vi "Main_Taper.vi"() -> ()   [LabVIEW 2016]
uses:
  <vilib>/Instr/_visa.llb/VISA Configure Serial Port (Instr).vi
panel:
  in  "Tab Control":T1(tab)=enum."Taper Time"
  in  "Stop Taper":bool
  out "COM_OK":bool
  in  "Send":bool
  in  "Start":bool
  in  "COM Write":string="AA;\nVL10.0000;\nAX;\nLS20;\nMR4.0000;\nGO;\nMR-4.0000;\nGO;\nLE;\nAA;\nVL1.0000,0.0800,0.0800;\nMR,-6.9491,-6.9491;\nGO;\nAX;\nLS11.0000;\nMR4.0000;\nGO;\nMR-4.0000\nGO;\nLE;"
  in  "COM Config":T2={"VISA resource name"="COM4", "baud rate"=9600, "data bits"=8, "parity"=enum."None", "stop bits"=10, "flow control"=0} {"flow control" items=["None"=0, "XON/XOFF"=1, "RTS/CTS"=2, "DTR/DSR"=4]; "data bits" min=5 max=8 step=1}
  in  "Stop Button":bool
  out "Taper Finish":bool
  in  "Diametro taper (um)":dbl=22.0
  in  "Longitud Cintura (mm)":dbl=8.0
  in  "Velocidad Estiramiento (mm/s)":dbl=0.08
  in  "Velocidad Quemador (mm/s)":dbl=1.0
  in  "Diametro inicial(um)":dbl=125.0
  out "Estiramiento (mm)":dbl=13.898170271551882
  out "Tiempo Requerido   (s)":dbl=102.86356419719925
  in  "Velocidad Precalentamiento (mm/s)":dbl=10.0 caption="Velocidad Precalentamiento"
  in  "Oscilaciones Precalentamiento":u8=20
  in  "Calcular movimiento":bool
  in  "Tiempo Estirameinto (s)":dbl=8.0
  in  "Longitud Cintura 2":dbl=8.0
  in  "Velocidad Estiramiento (mm/s) 2":dbl=0.08
  in  "Velocidad Quemador (mm/s) 2":dbl=1.0
  out "Estiramiento (mm) 2":dbl=13.898170271551882
  out "Tiempo Requerido   (s)  2":dbl=102.86356419719925
  in  "Velocidad Precalentamiento (mm/s) 2":dbl=10.0 caption="Velocidad Precalentamiento"
  in  "Oscilaciones Precalentamiento 2":u8=20 caption="Oscilaciones Precalentamiento"
  in  "Calcular movimiento 2":bool
  in  "SW_moveZ":bool
  in  "SW_moveY":bool
  in  "SW_moveX":bool
  in  "Velocidad Z":dbl
  in  "Velocidad Y":dbl
  in  "Velocidad X":dbl
  in  "Move Z":dbl
  in  "Move Y":dbl
  in  "Move X":dbl
  in  "Escribir Valores":bool
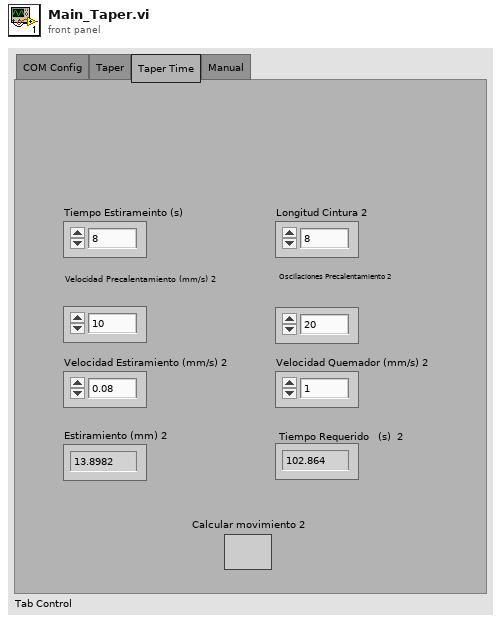
[diagram p1: front panel]
types:
  T1 = enum32{"COM Config", "Taper", "Taper Time", "Manual"}
  T2 = cluster{"VISA resource name":refnum<visa-resource-name>, "baud rate":u32, "data bits":u16, "parity":enum16{"None", "Odd", "Even", "Mark", "Space"}, "stop bits":u16, "flow control":u16}
  T3 = enum8{"Enabled", "Disabled", "Disabled and Grayed Out"}
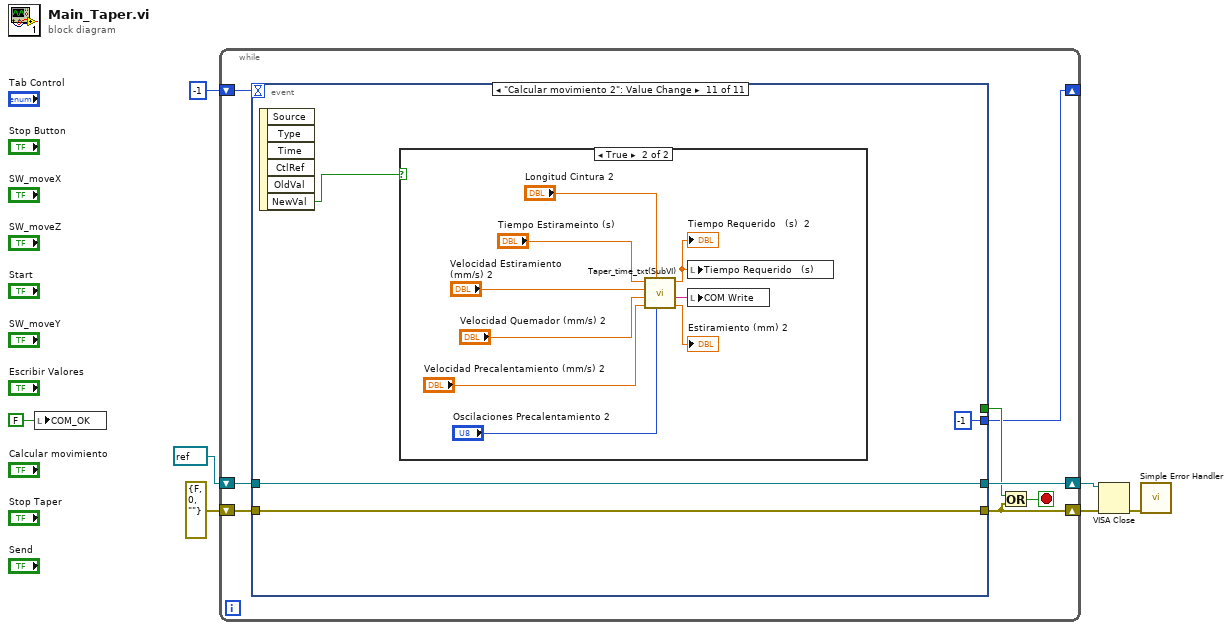
[diagram p0: block diagram]
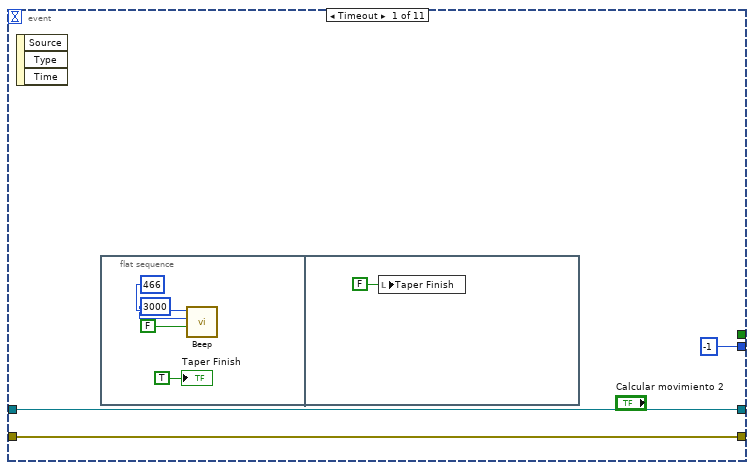
[diagram p2: hidden frame]
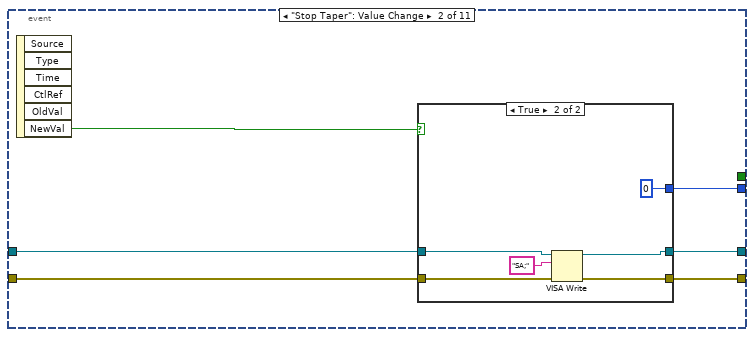
[diagram p3: hidden frame]
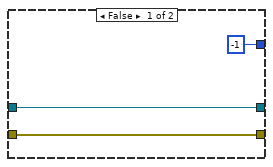
[diagram p4: hidden frame]
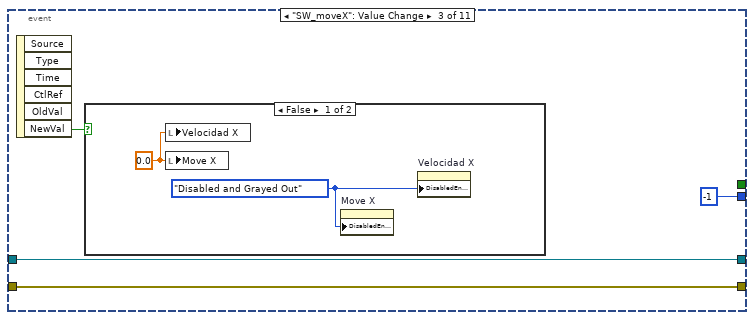
[diagram p5: hidden frame]
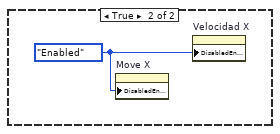
[diagram p6: hidden frame]
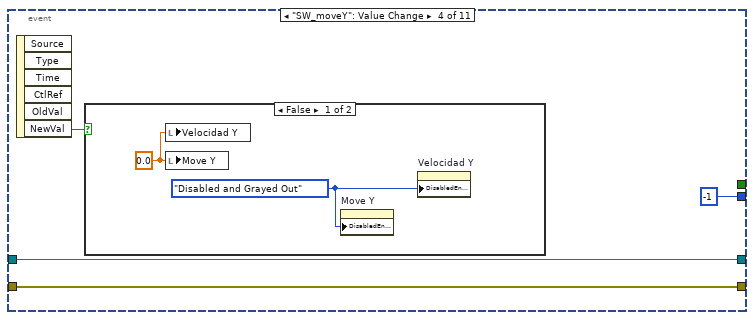
[diagram p7: hidden frame]
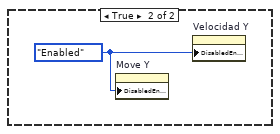
[diagram p8: hidden frame]
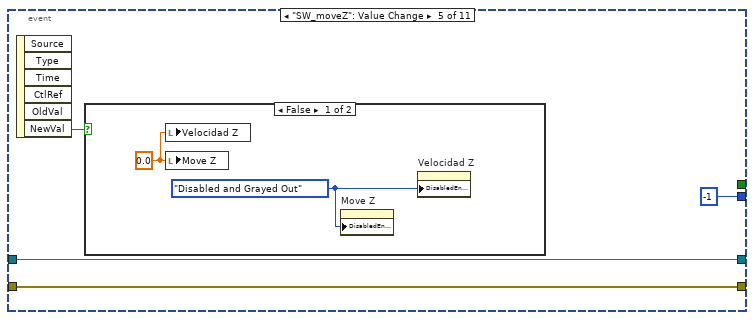
[diagram p9: hidden frame]
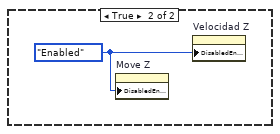
[diagram p10: hidden frame]
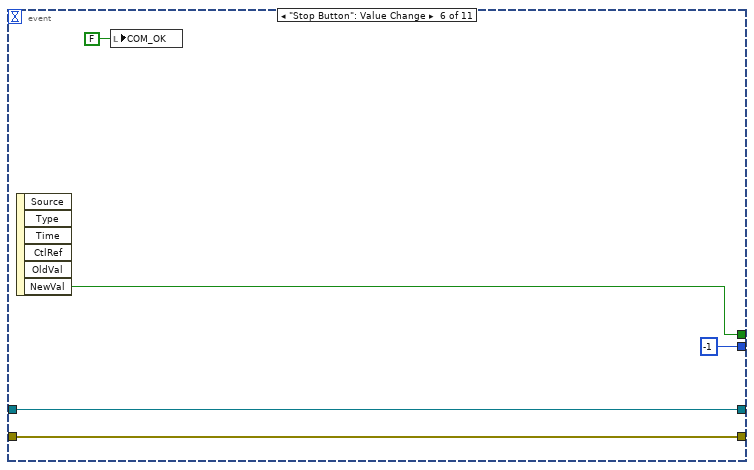
[diagram p11: hidden frame]
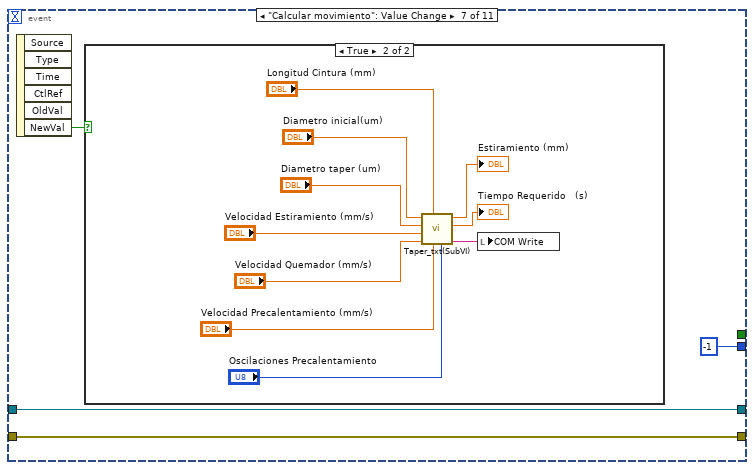
[diagram p12: hidden frame]
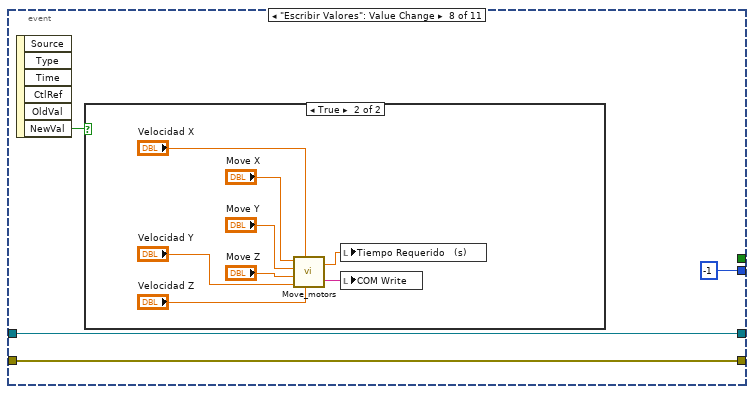
[diagram p14: hidden frame]
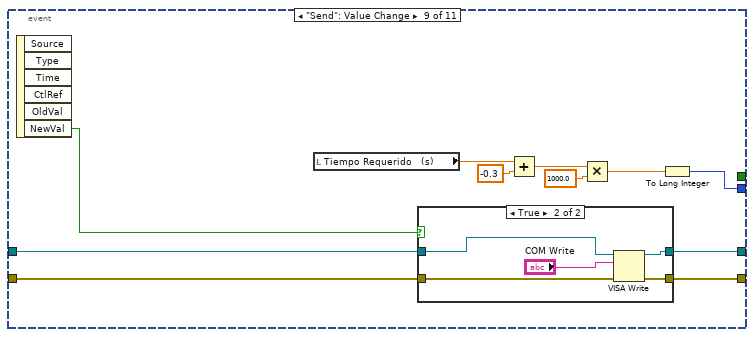
[diagram p16: hidden frame]
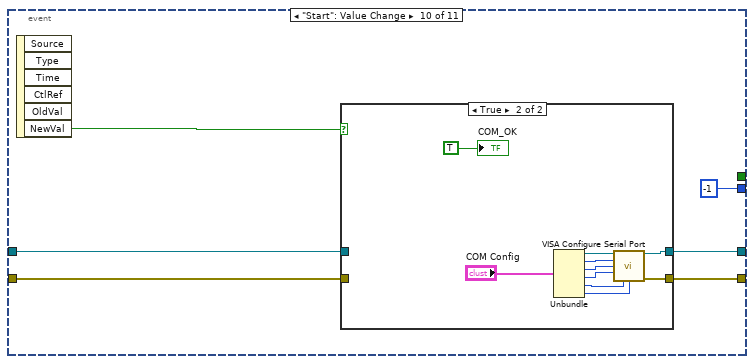
[diagram p18: hidden frame]
diagram:
  n1 = local write "COM_OK"(FALSE ("COM_OK")) -> ()
  n2 = while {
    shift-right: [w13] -> w7
    shift-left: refnum<visa-resource-name> refnum ("VISA resource name out") -> [w15]
    shift-right: [w10] -> w6
    shift-left: errorcluster {"status"=FALSE, "code"=0, "source"=""} ("error out") -> [w14]
    shift-right: [w9] -> _
    shift-left: -1 -> [w8]
    stop <- w11 stop-if-true
    n3 = event shown="[10] \"Calcular movimiento 2\": Value Change" {
      selector: _ -> [_ _ _ _ _ _ _ _ _ _ _]
      dyn-events: _ -> [_ _ _ _ _ _ _ _ _ _ _]
      timeout: w8 -> [_ _ _ _ _ _ _ _ _ _ _]
      tunnel: [w18 w24 w41 w48 w55 w64 w68 w81 w98 w113 w129] -> w13
      tunnel: [w17 w25 w40 w47 w54 w63 w67 w80 w97 w112 w128] -> w10
      tunnel: w15 -> [w18 w28 w41 w48 w55 w64 w68 w81 w100 w111 w129]
      tunnel: w14 -> [w17 w27 w40 w47 w54 w63 w67 w80 w99 w110 w128]
      tunnel: [_ _ _ _ _ w62 _ _ _ _ _] -> w12
      tunnel: [-1 w26 -1 -1 -1 -1 -1 -1 w91 -1 -1] -> w9
      event Timeout {
        n4 = event-data() -> ()  [unwired: 1 in, 3 out]
        n5 = flat-sequence {
          frame #0 {
            n6 = call <vilib>:"Beep.vi"("use system alert? (T)"=FALSE, "duration (msec)"=u32 3000, "frequency (Hz)"=u32 466) -> ()  [unwired: 9 in]
            "Taper Finish" <- TRUE ("Taper FInish")
          }
          frame #1 {
            n7 = local write "Taper Finish"(FALSE ("Taper FInish")) -> ()
          }
        }
      }
      event "Stop Taper": Value Change {
        n8 = event-data() -> ("NewVal"=w29:bool)  [unwired: 1 in, 5 out]
        n9 = case shown="True" w29 {
          tunnel: w28 -> [w32 w38]
          tunnel: w27 -> [w31 w37]
          tunnel: [w32 w36] -> w24
          tunnel: [w31 w35] -> w25
          tunnel: [-1 0] -> w26
          frame False {
          }
          frame True {
            n10 = VISA Write(VISA resource name=w38, write buffer="SA;", error in (no error)=w37) -> (VISA resource name out=w36:refnum<visa-resource-name>, error out=w35:errorcluster)  [unwired: 1 out]
          }
        }
      }
      event "SW_moveX": Value Change {
        n11 = event-data() -> ("NewVal"=w42:bool)  [unwired: 1 in, 5 out]
        n12 = case shown="False" w42 {
          frame False {
            w43 = T3."Disabled and Grayed Out" ("Disabled")
            w44 = 0.0 ("Move Z")
            n13 = local write "Velocidad X"(w44) -> ()
            n14 = local write "Move X"(w44) -> ()
            n15 = property on="Move X" class="DigNum (strict)"("DisabledEnum"=w43) -> ()  [unwired: 2 in, 2 out]
            n16 = property on="Velocidad X" class="DigNum (strict)"("DisabledEnum"=w43) -> ()  [unwired: 2 in, 2 out]
          }
          frame True {
            w45 = T3."Enabled" ("Disabled")
            n17 = property on="Move X" class="DigNum (strict)"("DisabledEnum"=w45) -> ()  [unwired: 2 in, 2 out]
            n18 = property on="Velocidad X" class="DigNum (strict)"("DisabledEnum"=w45) -> ()  [unwired: 2 in, 2 out]
          }
        }
      }
      event "SW_moveY": Value Change {
        n19 = event-data() -> ("NewVal"=w49:bool)  [unwired: 1 in, 5 out]
        n20 = case shown="False" w49 {
          frame False {
            w50 = 0.0 ("Move Z")
            w51 = T3."Disabled and Grayed Out" ("Disabled")
            n21 = local write "Velocidad Y"(w50) -> ()
            n22 = local write "Move Y"(w50) -> ()
            n23 = property on="Move Y" class="DigNum (strict)"("DisabledEnum"=w51) -> ()  [unwired: 2 in, 2 out]
            n24 = property on="Velocidad Y" class="DigNum (strict)"("DisabledEnum"=w51) -> ()  [unwired: 2 in, 2 out]
          }
          frame True {
            w52 = T3."Enabled" ("Disabled")
            n25 = property on="Move Y" class="DigNum (strict)"("DisabledEnum"=w52) -> ()  [unwired: 2 in, 2 out]
            n26 = property on="Velocidad Y" class="DigNum (strict)"("DisabledEnum"=w52) -> ()  [unwired: 2 in, 2 out]
          }
        }
      }
      event "SW_moveZ": Value Change {
        n27 = event-data() -> ("NewVal"=w56:bool)  [unwired: 1 in, 5 out]
        n28 = case shown="False" w56 {
          frame False {
            w57 = 0.0 ("Move Z")
            w58 = T3."Disabled and Grayed Out" ("Disabled")
            n29 = local write "Velocidad Z"(w57) -> ()
            n30 = local write "Move Z"(w57) -> ()
            n31 = property on="Move Z" class="DigNum (strict)"("DisabledEnum"=w58) -> ()  [unwired: 2 in, 2 out]
            n32 = property on="Velocidad Z" class="DigNum (strict)"("DisabledEnum"=w58) -> ()  [unwired: 2 in, 2 out]
          }
          frame True {
            w59 = T3."Enabled" ("Disabled")
            n33 = property on="Move Z" class="DigNum (strict)"("DisabledEnum"=w59) -> ()  [unwired: 2 in, 2 out]
            n34 = property on="Velocidad Z" class="DigNum (strict)"("DisabledEnum"=w59) -> ()  [unwired: 2 in, 2 out]
          }
        }
      }
      event "Stop Button": Value Change {
        n35 = event-data() -> ("NewVal"=w62:bool)  [unwired: 1 in, 5 out]
        n36 = local write "COM_OK"(FALSE ("COM_OK")) -> ()
      }
      event "Calcular movimiento": Value Change {
        n37 = event-data() -> ("NewVal"=w66:bool)  [unwired: 1 in, 5 out]
        n38 = case shown="True" w66 {
          frame False {
          }
          frame True {
            n39 = call "Taper_txt(SubVI).vi"("Oscilaciones Precalentamiento"="Oscilaciones Precalentamiento", "Velocidad Precalentamiento"="Velocidad Precalentamiento (mm/s)", "Longitud waist (mm)"="Longitud Cintura (mm)", "VELOCIDAD QUEMADOR (mm/s)"="Velocidad Quemador (mm/s)", "VELOCIDAD  STRETCHING"="Velocidad Estiramiento (mm/s)", "Diametro taper (um)"="Diametro taper (um)", "Diametro inicial(um)"="Diametro inicial(um)") -> ("COM Write"=w69:string, "TIEMPO REQUERIDO   (s)"=→"Tiempo Requerido   (s)":dbl, "Estiramiento (mm)"=→"Estiramiento (mm)":dbl)  [unwired: 2 in]
            n40 = local write "COM Write"(w69) -> ()
          }
        }
      }
      event "Escribir Valores": Value Change {
        n41 = event-data() -> ("NewVal"=w82:bool)  [unwired: 1 in, 5 out]
        n42 = case shown="True" w82 {
          frame False {
          }
          frame True {
            n43 = call "Move_motors.vi"("Velocidad Z"="Velocidad Z", "Velocidad X"="Velocidad X", "Velocidad Y"="Velocidad Y", "Move Z"="Move Z", "Move Y"="Move Y", "Move X"="Move X") -> ("COM Write"=w83:string, "Max Time"=w84:dbl)
            n44 = local write "Tiempo Requerido   (s)"(w84) -> ()
            n45 = local write "COM Write"(w83) -> ()
          }
        }
      }
      event "Send": Value Change {
        n46 = event-data() -> ("NewVal"=w101:bool)  [unwired: 1 in, 5 out]
        n47 = local read "Tiempo Requerido   (s)"() -> (w94:dbl)
        n48 = case shown="True" w101 {
          tunnel: w99 -> [w103 w107]
          tunnel: w100 -> [w102 w108]
          tunnel: [w102 w105] -> w98
          tunnel: [w103 w104] -> w97
          frame False {
          }
          frame True {
            n49 = VISA Write(VISA resource name=w108, write buffer="COM Write", error in (no error)=w107) -> (VISA resource name out=w105:refnum<visa-resource-name>, error out=w104:errorcluster)  [unwired: 1 out]
          }
        }
        n50 = Add(x=w94, y=-0.3) -> (x+y=w96:dbl)
        n51 = Multiply(x=w96, y=1000.0) -> (x*y=w93:dbl)
        n52 = To Long Integer(number=w93) -> (32bit integer=w91:i32)
      }
      event "Start": Value Change {
        n53 = event-data() -> ("NewVal"=w114:bool)  [unwired: 1 in, 5 out]
        n54 = case shown="True" w114 {
          tunnel: [w115 w119] -> w112
          tunnel: [w116 w118] -> w113
          tunnel: w111 -> [w116 _]
          tunnel: w110 -> [w115 _]
          frame False {
          }
          frame True {
            n55 = Unbundle("COM Config") -> ("VISA resource name"=w125:refnum<visa-resource-name>, "baud rate"=w124:u32, "data bits"=w123:u16, "parity"=w120:enum16{"None", "Odd", "Even", "Mark", "Space"}, "stop bits"=w122:u16, "flow control"=w121:u16)
            n56 = call-poly "VISA Configure Serial Port"("VISA resource name"=w125, "baud rate (9600)"=w124, "data bits (8)"=w123, "parity (0:none)"=w120, "stop bits (10: 1 bit)"=w122, "flow control (0:none)"=w121) -> ("VISA resource name out"=w118:refnum<visa-resource-name>, "error out"=w119:errorcluster)  [unwired: 8 in]
            "COM_OK" <- TRUE ("COM_OK")
          }
        }
      }
      event "Calcular movimiento 2": Value Change {
        n57 = event-data() -> ("NewVal"=w130:bool)  [unwired: 1 in, 5 out]
        n58 = case shown="True" w130 {
          frame False {
          }
          frame True {
            n59 = call "Taper_time_txt(SubVI).vi"("Oscilaciones Precalentamiento"="Oscilaciones Precalentamiento 2", "Longitud waist (mm)"="Longitud Cintura 2", "Velocidad Precalentamiento"="Velocidad Precalentamiento (mm/s) 2", "VELOCIDAD QUEMADOR (mm/s)"="Velocidad Quemador (mm/s) 2", "VELOCIDAD  STRETCHING"="Velocidad Estiramiento (mm/s) 2", "Tiempo Estiramiento (s)"="Tiempo Estirameinto (s)") -> ("Estiramiento (mm)"=→"Estiramiento (mm) 2":dbl, "COM Write"=w132:string, "TIEMPO REQUERIDO   (s)"=w131:dbl)  [unwired: 2 in]
            "Tiempo Requerido   (s)  2" <- w131
            n60 = local write "Tiempo Requerido   (s)"(w131) -> ()
            n61 = local write "COM Write"(w132) -> ()
          }
        }
      }
    }
    n62 = Or(x=w12, y=w10) -> (x .or. y?=w11:bool)
  }
  n63 = VISA Close(VISA resource name=w7, error in (no error)=w6) -> (error out=w5:errorcluster)
  n64 = call <vilib>:"Simple Error Handler.vi"("error in (no error)"=w5) -> ()  [unwired: 4 in, 5 out]
